vi "Instance to Map Entry.vi"(0 "MVA Comms VI in":refnum<class "Bind To Control Ref.lvclass">, 5 "Node Tests":refnum<class "Node Test.lvclass">[](array[class]), 11 "error in (no error)":errorcluster) -> (4 "MVA Comms VI out":refnum<class "Bind To Control Ref.lvclass">, 6 "Map Key":T2[](array[typedef]), 8 "Array":T1[](array[typedef]), 15 "error out":errorcluster)   [LabVIEW 2020, in "MVA Message Mapper.lvlib" / "Bind To Control Ref.lvclass"]
uses:
  <vilib>/gpm_packages/@cs/Bus-message-mapper/Source/support/Bind to Control Ref/Bind To Control Ref.lvclass
  C:/Program Files/National Instruments/LabVIEW 2020/vi.lib/gpm_packages/@cs/Bus-message-mapper/Source/support/MVA Comms/MVA Comms VI Instance.lvclass
  <vilib>/gpm_packages/@cs/Bus-message-mapper/Source/controls/Map Key.ctl
  <vilib>/gpm_packages/@cs/Bus-message-mapper/Source/controls/Datum Endpoint.ctl
  <vilib>/gpm_packages/@cs/Bus-message-mapper/Source/support/Traversal Algorithm/Node Test.lvclass
  <vilib>/gpm_packages/@cs/Bus-message-mapper/Source/support/MVA Comms/MVA Comms VI Instance.lvclass/MVA Comms VI Instance.ctl
  <vilib>/Utility/Data Type/Type Definitions/Data Type.ctl
  <vilib>/gpm_packages/@cs/Bus-message-mapper/Source/support/MVA Comms/Accessors/Read MVA Coms VI Instance.vi
  <vilib>/gpm_packages/@cs/Bus-message-mapper/Source/support/MVA Comms/Accessors/Read MVA Object In Terminal.vi
  <vilib>/gpm_packages/@cs/Bus-message-mapper/Source/support/MVA Comms/Accessors/Read Datum Value Terminal.vi
  <vilib>/gpm_packages/@cs/Bus-message-mapper/Source/support/MVA Comms/Accessors/Read Datum Name Terminal.vi
  <vilib>/gpm_packages/@cs/Bus-message-mapper/Source/support/MVA Comms/Accessors/Read MVA Coms VI Name.vi
  <vilib>/gpm_packages/@cs/Bus-message-mapper/Source/MVA Message Mapper.lvlib
  <vilib>/Utility/Data Type/NI_Data Type.lvlib
  <vilib>/gpm_packages/@cs/variant/Source/VariantExtensions.lvlib
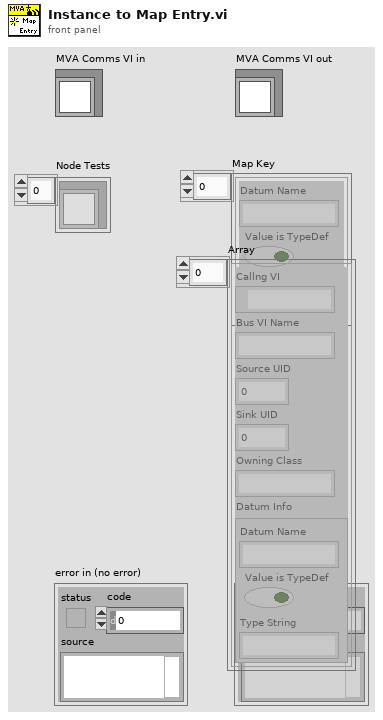
[diagram p1: front panel]
types:
  T1 = typedef "MVA Message Mapper.lvlib/Datum Endpoint.ctl" = cluster{"Callng VI":path, "Bus VI Name":string, "Source UID":i32, "Sink UID":i32, "Owning Class":string, "Datum Info":T2}
  T2 = typedef "MVA Message Mapper.lvlib/Map Key.ctl" = cluster{"Datum Name":string, "Value is TypeDef":bool, "Type String":string}
  T3 = typedef "NI_Data Type.lvlib/Data Type.ctl" = enum8{"Invalid Type", "Void", "I8", "I16", "I32", "I64", "U8", "U16", "U32", "U64", "Single Float", "Double Float", "Extended Float", "Single Complex", "Double Complex", "Extended Complex", "Enum U8", "Enum U16", "Enum U32", "Enum U64", "Single Float With Unit", "Double Float With Unit", "Extended Float With Unit", "Single Complex with Unit", "Double Complex with Unit", "Extended Complex with Unit", "Boolean", "String", "Path", "Picture", "Tag", "Array", "Cluster", "Variant", "LV Variant", "Waveform", "Timestamp", "Digital Waveform", "Digital Data", "ExpressData", "Refnum", "External Data", "VI", "Poly VI", "LabVIEW Class Instance", "Fixed Point", "Set Collection", "Map Collection"}
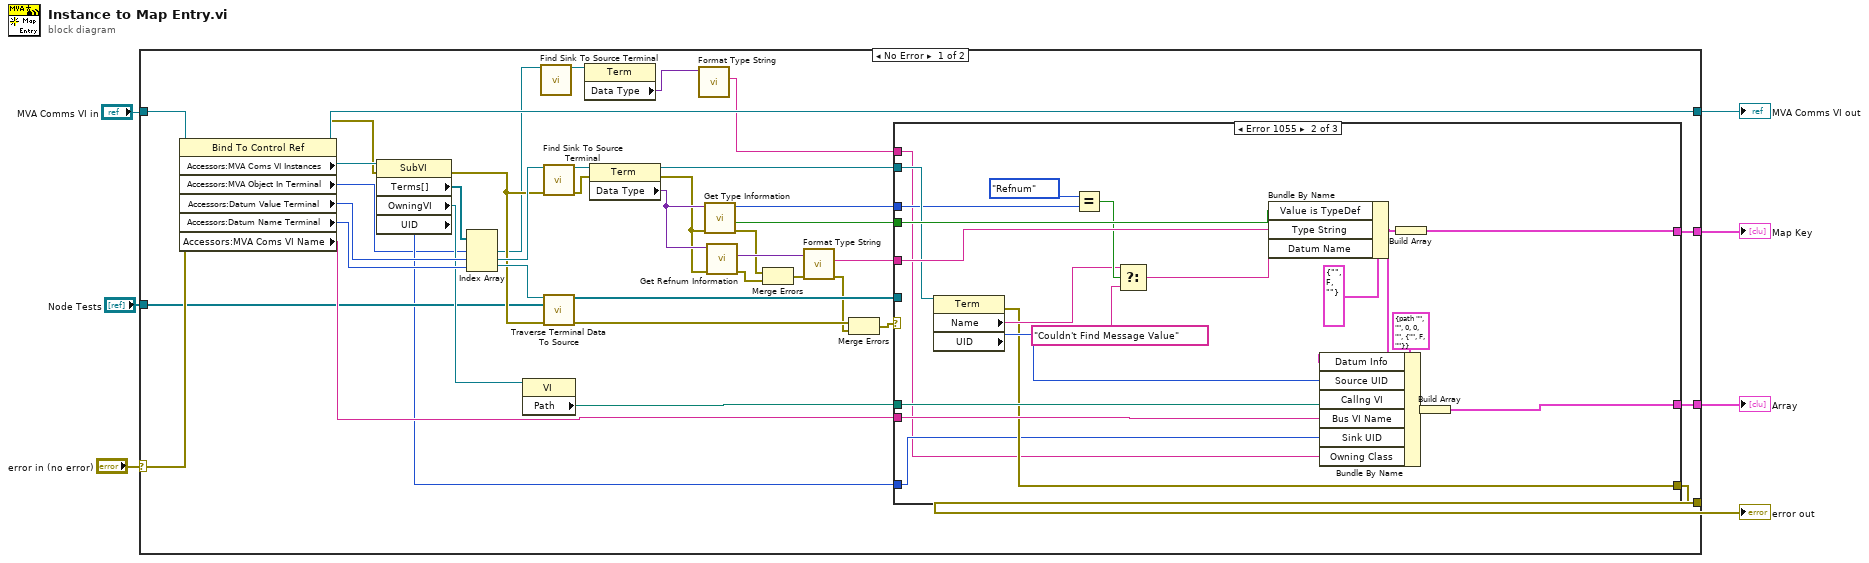
[diagram p0: block diagram]
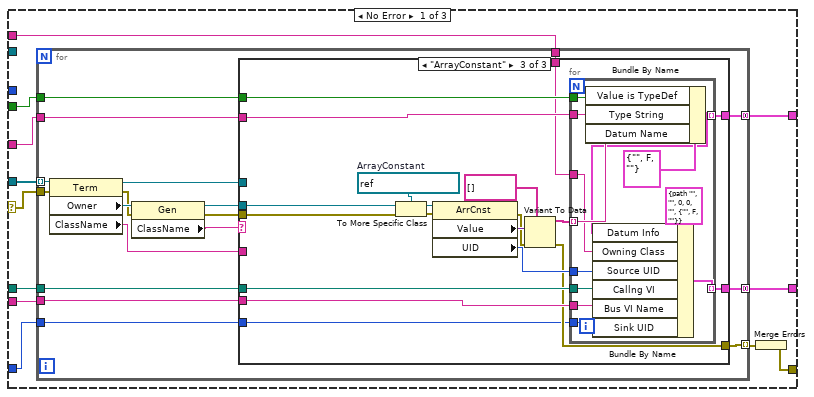
[diagram p2: hidden frame]
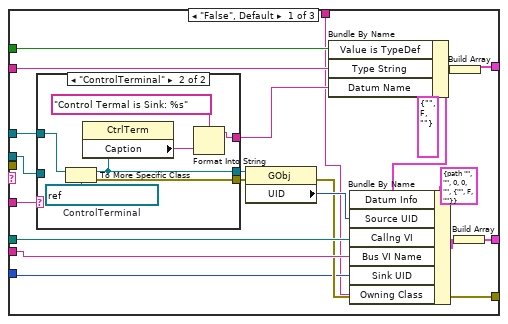
[diagram p3: hidden frame]
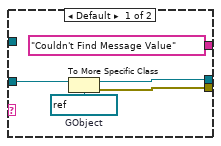
[diagram p4: hidden frame]
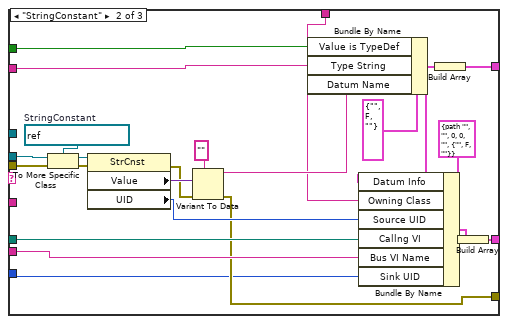
[diagram p5: hidden frame]
diagram:
  n1 = case shown="No Error" "error in (no error)" {
    selector: "error in (no error)" -> [w35 w187]
    tunnel: [w15 w187] -> w1
    tunnel: [w46 w186] -> w6
    tunnel: "MVA Comms VI in" -> [w47 w186]
    tunnel: [w40 _] -> w4
    tunnel: "Node Tests" -> [w29 _]
    tunnel: [w28 _] -> w3
    frame No Error {
      n2 = property class="Bind To Control Ref"(reference=w47, error in=w35) -> (reference out=w46:refnum<class "Bind To Control Ref.lvclass">, error out=w34:errorcluster, "Accessors:MVA Coms VI Instances"=w43:refnum<vi>, "Accessors:MVA Object In Terminal"=w10:i32, "Accessors:Datum Value Terminal"=w42:i32, "Accessors:Datum Name Terminal"=w41:i32, "Accessors:MVA Coms VI Name"=w37:string)
      n3 = property class="SubVI"(reference=w43, error in=w34) -> (error out=w31:errorcluster, "Terms[]"=w45:refnum<vi>[], "OwningVI"=w38:refnum<vi>, "UID"=w14:i32)  [unwired: 1 out]
      n4 = Index Array(array=w45, index #1=w10, index #2=w42, index #3=w41) -> (element #1=w9:refnum<vi>, element #2=w33:refnum<vi>, element #3=w44:refnum<vi>)
      n5 = property class="VI"(reference=w38) -> ("Path"=w36:path)  [unwired: 1 in, 2 out]
      n6 = call <vilib>:"Find Sink To Source Terminal.vi"("Source Terminal"=w9) -> ("Sink Terminal"=w12:refnum<vi>)  [unwired: 13 in, 1 out]
      n7 = call <vilib>:"Find Sink To Source Terminal.vi"("Source Terminal"=w33, "error in (no error)"=w31) -> ("Sink Terminal"=w13:refnum<vi>, "error out"=w30:errorcluster)  [unwired: 12 in]
      n8 = call <vilib>:"Traverse Terminal Data To Source.vi"("Terminal in"=w44, "Node Tests"=w29, "error in (no error)"=w31) -> ("Source Terminals"=w39:refnum<vi>[], "error out"=w18:errorcluster)  [unwired: 11 in]
      n9 = property on="Property Node" class="Term"(reference=w12) -> ("Data Type"=w11:variant)  [unwired: 1 in, 2 out]
      n10 = property on="Property Node" class="Term"(reference=w13, error in=w30) -> (reference out=w25:refnum<vi>, error out=w23:errorcluster, "Data Type"=w27:variant)
      n11 = call <vilib>:"Format Type String.vi"("Data Type"=w11) -> ("Type Name"=w8:string)  [unwired: 9 in, 1 out]
      n12 = call <vilib>:"Get Type Information.vi"("error in (no error)"=w23, "variant"=w27) -> ("error out"=w19:errorcluster, "type definition"=w32:bool, "type"=w22:T3)  [unwired: 5 in, 2 out]
      n13 = call <vilib>:"Get Refnum Information.vi"("error in (no error)"=w23, "variant"=w27) -> ("error out"=w20:errorcluster, "strict type"=w24:variant)  [unwired: 6 in, 2 out]
      n14 = Merge Errors(w19, w20) -> (w21:errorcluster)
      n15 = call <vilib>:"Format Type String.vi"("error in (no error)"=w21, "Data Type"=w24) -> ("error out"=w17:errorcluster, "Type Name"=w26:string)  [unwired: 8 in]
      n16 = Merge Errors(w18, w17) -> (w16:errorcluster)
      n17 = case shown="Error 1055" w16 {
        selector: w16 -> [w52 _ w185]
        tunnel: [w59 w178 _] -> w40
        tunnel: w39 -> [w58 _ _]
        tunnel: w37 -> [w57 w181 _]
        tunnel: w36 -> [w56 w182 _]
        tunnel: w32 -> [w55 w184 _]
        tunnel: [w54 w177 _] -> w28
        tunnel: w26 -> [w53 w183 _]
        tunnel: w25 -> [_ w180 _]
        tunnel: w22 -> [_ w172 _]
        tunnel: [w51 w167 w185] -> w15
        tunnel: w14 -> [w49 w166 _]
        tunnel: w8 -> [w48 w165 _]
        frame No Error {
          n18 = for {
            tunnel: [w70] -> w59 mode=concatenating
            tunnel: w58 -> [w76] mode=indexing
            tunnel: w57 -> [w68]
            tunnel: w56 -> [w69]
            tunnel: w55 -> [w72]
            tunnel: w53 -> [w71]
            tunnel: [w67] -> w54 mode=concatenating
            tunnel: w52 -> [w66]
            tunnel: [w64] -> w50 mode=indexing
            tunnel: w49 -> [w63]
            tunnel: w48 -> [w60]
            n19 = property on="Property Node" class="Term"(reference=w76, error in=w66) -> (reference out=w62:refnum<vi>, error out=w74:errorcluster, "Owner"=w77:refnum<vi>, "ClassName"=w61:string)
            n20 = property on="Property Node" class="Gen"(reference=w77, error in=w74) -> (reference out=w73:refnum<vi>, error out=w65:errorcluster, "ClassName"=w75:string)
            n21 = case shown="\"ArrayConstant\"" w75 {
              tunnel: w73 -> [w84 w128 w148]
              tunnel: w72 -> [w95 w125 w146]
              tunnel: w71 -> [w96 w126 w145]
              tunnel: [w94 w123 w143] -> w70
              tunnel: w69 -> [w91 w120 w142]
              tunnel: w68 -> [w90 w119 w141]
              tunnel: [w88 w117 w139] -> w67
              tunnel: w65 -> [_ w116 w138]
              tunnel: [w87 w113 w135] -> w64
              tunnel: w63 -> [w86 w112 w134]
              tunnel: w62 -> [w85 _ _]
              tunnel: w61 -> [w80 _ _]
              tunnel: w60 -> [w79 w111 w133]
              frame "False", Default {
                n22 = case shown="\"ControlTerminal\"" w80 {
                  tunnel: [w102 w104] -> w82
                  tunnel: w84 -> [w100 _]
                  tunnel: [w99 w107] -> w81
                  tunnel: w85 -> [_ w108]
                  tunnel: ["Couldn't Find Message Value" w105] -> w83
                  frame Default {
                    w101 = refnum<vi> refnum  # GObject
                    n23 = To More Specific Class(target class=w101, reference=w100) -> (specific class reference=w102:refnum<vi>, error out=w99:errorcluster)  [unwired: 1 in]
                  }
                  frame "ControlTerminal" {
                    w109 = refnum<vi> refnum  # ControlTerminal
                    n24 = To More Specific Class(target class=w109, reference=w108) -> (specific class reference=w104:refnum<vi>, error out=w107:errorcluster)  [unwired: 1 in]
                    n25 = property on="Property Node" class="CtrlTerm"(reference=w104) -> ("Caption"=w103:string)  [unwired: 1 in, 2 out]
                    n26 = Format Into String(format string="Control Termal is Sink: %s", w103) -> (resulting string=w105:string)  [unwired: 2 in, 1 out]
                  }
                }
                n27 = property class="GObj"(reference=w82, error in=w81) -> (error out=w87:errorcluster, "UID"=w92:i32)  [unwired: 1 out]
                n28 = Bundle By Name(cluster=T2 {"Datum Name"="", "Value is TypeDef"=FALSE, "Type String"=""} ("Map Key"), "Value is TypeDef"=w95, "Type String"=w96, "Datum Name"=w83) -> (w78:T2)
                n29 = Bundle By Name(cluster=T1 {"Callng VI"=path "", "Bus VI Name"="", "Source UID"=0, "Sink UID"=0, "Owning Class"="", "Datum Info"={"Datum Name"="", "Value is TypeDef"=FALSE, "Type String"=""}} ("Set Value"), "Datum Info"=w78, "Source UID"=w92, "Callng VI"=w91, "Bus VI Name"=w90, "Sink UID"=w86, "Owning Class"=w79) -> (w89:T1)
                n30 = Build Array(w78) -> (w94:T2[])
                n31 = Build Array(w89) -> (w88:T1[])
              }
              frame "StringConstant" {
                w132 = refnum<vi> refnum  # StringConstant
                n32 = To More Specific Class(target class=w132, reference=w128, error in=w116) -> (specific class reference=w131:refnum<vi>, error out=w115:errorcluster)
                n33 = property class="StrCnst"(reference=w131, error in=w115) -> (error out=w114:errorcluster, "Value"=w130:variant, "UID"=w121:i32)  [unwired: 1 out]
                n34 = Variant To Data(error in=w114, type="", Variant=w130) -> (data=w127:string, error out=w113:errorcluster)
                n35 = Bundle By Name(cluster=T2 {"Datum Name"="", "Value is TypeDef"=FALSE, "Type String"=""} ("Map Key"), "Value is TypeDef"=w125, "Type String"=w126, "Datum Name"=w127) -> (w110:T2)
                n36 = Bundle By Name(cluster=T1 {"Callng VI"=path "", "Bus VI Name"="", "Source UID"=0, "Sink UID"=0, "Owning Class"="", "Datum Info"={"Datum Name"="", "Value is TypeDef"=FALSE, "Type String"=""}} ("Set Value"), "Datum Info"=w110, "Owning Class"=w111, "Source UID"=w121, "Callng VI"=w120, "Bus VI Name"=w119, "Sink UID"=w112) -> (w118:T1)
                n37 = Build Array(w110) -> (w123:T2[])
                n38 = Build Array(w118) -> (w117:T1[])
              }
              frame "ArrayConstant" {
                w151 = refnum<vi> refnum  # ArrayConstant
                n39 = To More Specific Class(target class=w151, reference=w148, error in=w138) -> (specific class reference=w150:refnum<vi>, error out=w137:errorcluster)
                n40 = property class="ArrCnst"(reference=w150, error in=w137) -> (error out=w136:errorcluster, "Value"=w149:variant, "UID"=w140:i32)  [unwired: 1 out]
                n41 = Variant To Data(error in=w136, type=string[] [], Variant=w149) -> (data=w144:string[], error out=w135:errorcluster)
                n42 = for {
                  tunnel: w146 -> [w162]
                  tunnel: w145 -> [w161]
                  tunnel: w144 -> [w160] mode=indexing
                  tunnel: [w152] -> w143 mode=indexing
                  tunnel: w142 -> [w158]
                  tunnel: w141 -> [w157]
                  tunnel: w140 -> [w156]
                  tunnel: [w155] -> w139 mode=indexing
                  tunnel: w134 -> [w154]
                  tunnel: w133 -> [w153]
                  n43 = Bundle By Name(cluster=T2 {"Datum Name"="", "Value is TypeDef"=FALSE, "Type String"=""} ("Map Key"), "Value is TypeDef"=w162, "Type String"=w161, "Datum Name"=w160) -> (w152:T2)
                  n44 = Bundle By Name(cluster=T1 {"Callng VI"=path "", "Bus VI Name"="", "Source UID"=0, "Sink UID"=0, "Owning Class"="", "Datum Info"={"Datum Name"="", "Value is TypeDef"=FALSE, "Type String"=""}} ("Set Value"), "Datum Info"=w152, "Owning Class"=w153, "Source UID"=w156, "Callng VI"=w158, "Bus VI Name"=w157, "Sink UID"=w154) -> (w155:T1)
                }
              }
            }
          }
          n45 = Merge Errors(w50) -> (w51:errorcluster)
        }
        frame Error {
          n46 = property on="Property Node" class="Term"(reference=w180) -> (error out=w167:errorcluster, "Name"=w170:string, "UID"=w179:i32)  [unwired: 1 in, 1 out]
          n47 = Equal?(x=Data_Type."Refnum" ("y"), y=w172) -> (x = y?=w171:bool)
          n48 = Select(t=w170, s=w171, f="Couldn't Find Message Value") -> (s? t:f=w173:string)
          n49 = Bundle By Name(cluster=T2 {"Datum Name"="", "Value is TypeDef"=FALSE, "Type String"=""} ("Map Key"), "Value is TypeDef"=w184, "Type String"=w183, "Datum Name"=w173) -> (w164:T2)
          n50 = Bundle By Name(cluster=T1 {"Callng VI"=path "", "Bus VI Name"="", "Source UID"=0, "Sink UID"=0, "Owning Class"="", "Datum Info"={"Datum Name"="", "Value is TypeDef"=FALSE, "Type String"=""}} ("Set Value"), "Datum Info"=w164, "Source UID"=w179, "Callng VI"=w182, "Bus VI Name"=w181, "Sink UID"=w166, "Owning Class"=w165) -> (w174:T1)
          n51 = Build Array(w164) -> (w178:T2[])
          n52 = Build Array(w174) -> (w177:T1[])
        }
        frame Default {
        }
      }
    }
    frame Error {
    }
  }
  "error out" <- w1
  "MVA Comms VI out" <- w6
  "Map Key" <- w4
  "Array" <- w3
